vi "ActionVIOnCompile.vi"(8 "error in (no error)":errorcluster, 11 "Device Item Ref in":T1 format="%.0x") -> (0 "error out":errorcluster)   [LabVIEW 2023, in "Embedded TDMS Logger System Explorer.lvlib"]
uses:
  Embedded TDMS Logger System Explorer.lvlib
  <vilib>/NI VeriStand/Custom Device API/Custom Device Item Ref.ctl
  Shared/Compiled.Settings.ctl
  Shared/FileData.ctl
  Shared/GroupData.ctl
  Shared/Meta Data Item.ctl
  Shared/ChannelData.ctl
  <vilib>/NI VeriStand/Custom Device API/Data Reference.ctl
  Shared/SegmentOptions.ctl
  <vilib>/NI VeriStand/Custom Device API/Custom Device Channel Type.ctl
  <vilib>/NI VeriStand/Custom Device API/Get Item Property (U16).vi
  <vilib>/NI VeriStand/Custom Device API/Get Item Property (Variant).vi
  <vilib>/NI VeriStand/Custom Device API/Get Item Property (Dependent Node Pointer).vi
  <vilib>/NI VeriStand/Custom Device API/Get Item Property (Boolean).vi
  <vilib>/NI VeriStand/Custom Device API/Get Item Property (String).vi
  <vilib>/NI VeriStand/Custom Device API/Get Item Property (Double).vi
  <vilib>/NI VeriStand/Custom Device API/Set Item Property (Variant).vi
  <vilib>/NI VeriStand/Custom Device API/Custom Device API.lvlib
  <vilib>/NI/NIVS Inline Async API/_Data Access System Explorer/Data Access System Explorer.lvlib
  Shared/Embedded TDMS Logger Shared.lvlib
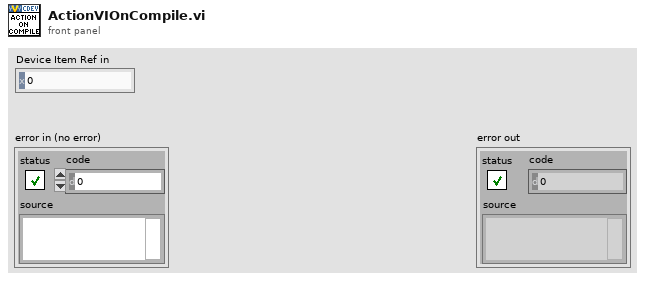
[diagram p1: front panel]
types:
  T1 = typedef "Custom Device API.lvlib/Custom Device Item Ref.ctl" = u64
  T2 = cluster{"Name":string, "Type":enum16{"Output/Write", "Input/Read", "Input/ReadWrite"}, "VS Refs":T1[]}
  T3 = enum16{"Output/Write", "Input/Read", "Input/ReadWrite"}
  T4 = typedef "Custom Device API.lvlib/Custom Device Channel Type.ctl" = enum16{"Input", "Output"}
  T5 = typedef "Embedded TDMS Logger Shared.lvlib/FileData.ctl" = cluster{"Date Captured":string, "Directory":string, "Name":string, "Groups":T6[], "Meta Data":T7[]}
  T6 = typedef "Embedded TDMS Logger Shared.lvlib/GroupData.ctl" = cluster{"Data Rate":string, "Meta Data":T7[], "Channels":T8[], "Name":string}
  T7 = typedef "Embedded TDMS Logger Shared.lvlib/Meta Data Item.ctl" = cluster{"Key":string, "Value":string}
  T8 = typedef "Embedded TDMS Logger Shared.lvlib/ChannelData.ctl" = cluster{"Name":string, "Meta Data":T7[], "Data Reference":T9, "Wfm?":bool, "Increment":dbl}
  T9 = typedef "Custom Device API.lvlib/Data Reference.ctl" = i32
  T10 = typedef "Embedded TDMS Logger Shared.lvlib/Compiled.Settings.ctl" = cluster{"Name":string, "Async Init Timeout":u16, "File Data":T5, "Segment Files":bool, "Segment Every":dbl, "Trigger?":bool, "Segment by":T11, "Trigger Ref":T9}
  T11 = typedef "SegmentOptions.ctl" = enum16{"Time (s)", "Size (MB)"}
  T12 = typedef "Custom Device API.lvlib/Custom Device Item Info.ctl" = cluster{"Name":string, "Is Channel":bool, "GUID":string, "Is Waveform":bool}
  T13 = typedef "Custom Device API.lvlib/Waveform Data Reference.ctl" = i32
  T14 = cluster{"Name":string, "Type":enum16{"Output/Write", "Input/Read", "Input/ReadWrite"}, "VS Refs":T1[]}[]
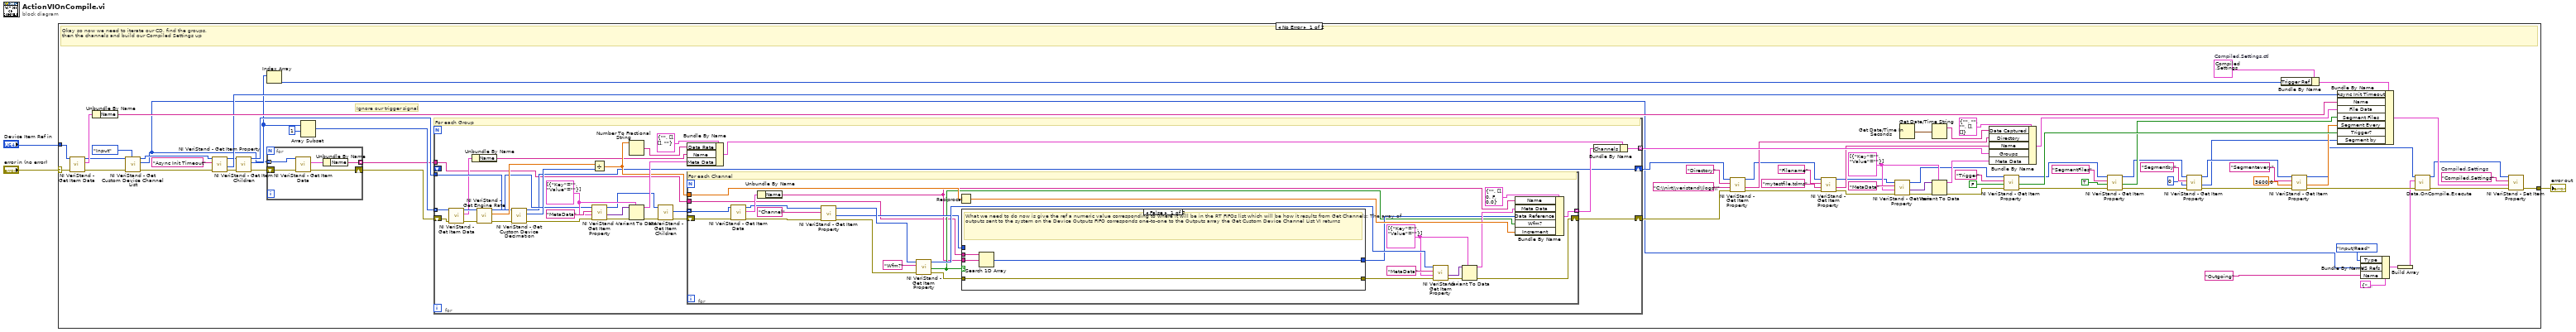
[diagram p0: block diagram]
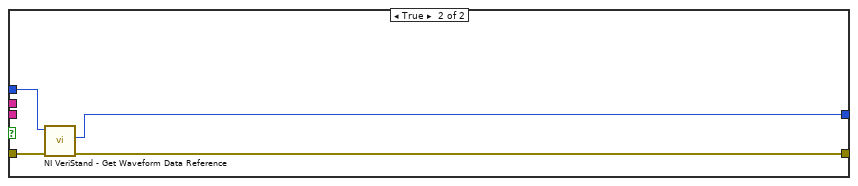
[diagram p2: hidden frame]
diagram:
  n1 = case shown="No Error" "error in (no error)" {
    selector: "error in (no error)" -> [w78 w152]
    tunnel: [w79 w152] -> w2
    tunnel: "Device Item Ref in" -> [w65 _]
    frame No Error {
      w42 = T7[] [{"Key"="", "Value"=""}]
      w50 = T10 {"Name"="", "Async Init Timeout"=0, "File Data"={"Date Captured"="", "Directory"="", "Name"="", "Groups"=[], "Meta Data"=[]}, "Segment Files"=FALSE, "Segment Every"=0.0, "Trigger?"=FALSE, "Segment by"=enum."Size (MB)", "Trigger Ref"=0}  # Compiled.Settings.ctl
      w81 = "Compiled.Settings"  # Compiled.Settings
      # "Ignore our trigger signal"
      # "Okay so now we need to iterate our CD, find the groups,\nthen the channels and build our Compiled Settings up"
      n2 = call <vilib>:"NI VeriStand - Get Item Data.vi"("error in (no error)"=w78, "Item Ref in"=w65) -> ("error out"=w17:errorcluster, "Item Info"=w77:T12, "Item Ref out"=w18:T1)  [unwired: 6 in, 1 out]
      n3 = Unbundle By Name(w77) -> ("Name"=w76:string)
      n4 = call <vilib>:"NI VeriStand - Get Custom Device Channel List.vi"("Channel Type"=Custom_Device_Channel_Type."Input", "error in (no error)"=w17, "Device Ref in"=w18) -> ("error out"=w16:errorcluster, "Specified Channel Ref List"=w7:T1[], "Device Ref out"=w15:T1)  [unwired: 6 in]
      n5 = call-poly <vilib>:"NI VeriStand - Get Item Property.vi"("error in (no error)"=w16, "Property Name"="Async Init Timeout", "Item Ref in"=w15) -> ("error out"=w71:errorcluster, "Value"=w72:u16, "Item Ref out"=w58:T1)  [unwired: 5 in, 1 out]
      n6 = call <vilib>:"NI VeriStand - Get Item Children.vi"("error in (no error)"=w71, "Item Ref in"=w58) -> ("error out"=w13:errorcluster, "Child Refs"=w51:T1[], "Item Ref out"=w56:T1)  [unwired: 6 in, 1 out]
      n7 = Index Array(array=w51) -> (element=w49:T1)  [unwired: 1 in]
      n8 = for {
        tunnel: w7 -> [w86] mode=indexing
        tunnel: [w84] -> w14 mode=indexing
        shift-right: [w83] -> w12
        shift-left: w13 -> [w82]
        n9 = call <vilib>:"NI VeriStand - Get Item Data.vi"("error in (no error)"=w82, "Item Ref in"=w86) -> ("error out"=w83:errorcluster, "Item Info"=w85:T12)  [unwired: 8 out]
        n10 = Unbundle By Name(w85) -> ("Name"=w84:string)
      }
      n11 = Array Subset(array=w51, index=1 ("length")) -> (w55:T1[])  [unwired: 1 in]
      n12 = for {
        tunnel: w55 -> [w94] mode=indexing
        shift-right: [w97] -> w60
        shift-left: w12 -> [w93]
        tunnel: [w115] -> w69 mode=indexing
        tunnel: w56 -> [w107]
        shift-right: [w88] -> w59
        shift-left: _ -> [_]
        tunnel: w14 -> [w87]
        w104 = T7[] [{"Key"="", "Value"=""}]
        # "For each Group"
        n13 = call <vilib>:"NI VeriStand - Get Item Data.vi"("error in (no error)"=w93, "Item Ref in"=w94) -> ("error out"=w92:errorcluster, "Item Info"=w90:T12, "Item Ref out"=w91:T1)  [unwired: 7 out]
        n14 = Unbundle By Name(w90) -> ("Name"=w89:string)
        n15 = call <vilib>:"NI VeriStand - Get Engine Rate.vi"("error in (no error)"=w92, "Item Ref in"=w91) -> ("error out"=w108:errorcluster, "Rate (Hz)"=w111:dbl, "Item Ref out"=w96:T1)  [unwired: 7 in]
        n16 = call <vilib>:"NI VeriStand - Get Custom Device Decimation.vi"("error in (no error)"=w108, "Device Ref in"=w107) -> ("error out"=w102:errorcluster, "Decimation"=w110:i32, "Device Ref out"=w88:T1)  [unwired: 7 in]
        n17 = Divide(x=w111, y=w110) -> (x/y=w99:dbl)
        n18 = call-poly <vilib>:"NI VeriStand - Get Item Property.vi"("error in (no error)"=w102, "Default Value"=w104, "Property Name"="MetaData", "Item Ref in"=w96) -> ("error out"=w101:errorcluster, "Value"=w105:variant, "Item Ref out"=w95:T1)  [unwired: 4 in, 1 out]
        n19 = Number To Fractional String(number=w99) -> (F-format string=w109:string)  [unwired: 3 in]
        n20 = Variant To Data(error in=w101, type=w104, Variant=w105) -> (data=w103:T7[], error out=w100:errorcluster)
        n21 = call <vilib>:"NI VeriStand - Get Item Children.vi"("error in (no error)"=w100, "Item Ref in"=w95) -> ("error out"=w98:errorcluster, "Child Refs"=w112:T1[])  [unwired: 6 in, 2 out]
        n22 = Bundle By Name(cluster=T6 {"Data Rate"="", "Meta Data"=[], "Channels"=[], "Name"=""} ("Group Data"), "Data Rate"=w109, "Name"=w89, "Meta Data"=w103) -> (w113:T6)
        n23 = for {
          tunnel: [w142] -> w116 mode=indexing
          tunnel: w112 -> [w125] mode=indexing
          tunnel: w99 -> [w140]
          shift-right: [w129] -> w97
          shift-left: w98 -> [w124]
          tunnel: w87 -> [w117]
          w131 = T7[] [{"Key"="", "Value"=""}]
          # "For each Channel"
          n24 = call <vilib>:"NI VeriStand - Get Item Data.vi"("error in (no error)"=w124, "Item Ref in"=w125) -> ("error out"=w128:errorcluster, "Item Info"=w127:T12, "Item Ref out"=w126:T1)  [unwired: 7 out]
          n25 = Unbundle By Name(w127) -> ("Name"=w118:string)
          n26 = call-poly <vilib>:"NI VeriStand - Get Item Property.vi"("error in (no error)"=w128, "Property Name"="Channel", "Item Ref in"=w126) -> ("error out"=w136:errorcluster, "Dependent Node Ref"=w123:T1, "Item Ref out"=w137:T1)  [unwired: 5 in, 1 out]
          n27 = call-poly <vilib>:"NI VeriStand - Get Item Property.vi"("error in (no error)"=w136, "Property Name"="Wfm?", "Item Ref in"=w137) -> ("error out"=w122:errorcluster, "Value"=w119:bool, "Item Ref out"=w134:T1)  [unwired: 5 in, 1 out]
          n28 = Reciprocal(x=w140) -> (1/x=w141:dbl)
          n29 = case shown="False" w119 {
            tunnel: w123 -> [_ w151]
            tunnel: w122 -> [w147 w150]
            tunnel: [w147 w149] -> w121
            tunnel: [w144 w148] -> w120
            tunnel: w118 -> [w146 _]
            tunnel: w117 -> [w145 _]
            frame False {
              # "What we need to do now is give the ref a numeric value corresponding to where it will be in the RT FIFOs list which will be how it results from Get Channels: The array of outputs sent to the system on the Device Outputs FIFO corresponds one-to-one to the Outputs array the Get Custom Device Channel List VI returns"
              n30 = Search 1D Array(1D array=w145, element=w146) -> (index of element=w144:i32)  [unwired: 1 in]
            }
            frame True {
              n31 = call <vilib>:"NI VeriStand - Get Waveform Data Reference.vi"("error in (no error)"=w150, "Waveform Ref in"=w151) -> ("error out"=w149:errorcluster, "Waveform Data Reference"=w148:T13)  [unwired: 7 in, 1 out]
            }
          }
          n32 = call-poly <vilib>:"NI VeriStand - Get Item Property.vi"("error in (no error)"=w121, "Default Value"=w131, "Property Name"="MetaData", "Item Ref in"=w134) -> ("error out"=w133:errorcluster, "Value"=w132:variant)  [unwired: 4 in, 2 out]
          n33 = Variant To Data(error in=w133, type=w131, Variant=w132) -> (data=w130:T7[], error out=w129:errorcluster)
          n34 = Bundle By Name(cluster=T8 {"Name"="", "Meta Data"=[], "Data Reference"=0, "Wfm?"=FALSE, "Increment"=0.0} ("Channel Data"), "Name"=w118, "Meta Data"=w130, "Data Reference"=w120, "Wfm?"=w119, "Increment"=w141) -> (w142:T8)
        }
        n35 = Bundle By Name(cluster=w113, "Channels"=w116) -> (w115:T6)
      }
      n36 = call-poly <vilib>:"NI VeriStand - Get Item Property.vi"("error in (no error)"=w60, "Default Value"="C:\\nirt\\veristand\\logs\\", "Property Name"="Directory", "Item Ref in"=w59) -> ("error out"=w46:errorcluster, "Value"=w64:string, "Item Ref out"=w61:T1)  [unwired: 4 in, 1 out]
      n37 = call-poly <vilib>:"NI VeriStand - Get Item Property.vi"("error in (no error)"=w46, "Default Value"="mytestfile.tdms", "Property Name"="Filename", "Item Ref in"=w61) -> ("error out"=w44:errorcluster, "Value"=w57:string, "Item Ref out"=w41:T1)  [unwired: 4 in, 1 out]
      n38 = call-poly <vilib>:"NI VeriStand - Get Item Property.vi"("error in (no error)"=w44, "Default Value"=w42, "Property Name"="MetaData", "Item Ref in"=w41) -> ("error out"=w43:errorcluster, "Value"=w45:variant, "Item Ref out"=w37:T1)  [unwired: 4 in, 1 out]
      n39 = Get Date/Time In Seconds() -> (seconds since 1Jan1904=w53:timestamp)
      n40 = Get Date/Time String(seconds (now)=w53) -> (date string=w52:string)  [unwired: 2 in, 1 out]
      n41 = Variant To Data(error in=w43, type=w42, Variant=w45) -> (data=w40:T7[], error out=w36:errorcluster)
      n42 = Bundle By Name(cluster=T5 {"Date Captured"="", "Directory"="", "Name"="", "Groups"=[], "Meta Data"=[]} ("File Data"), "Date Captured"=w52, "Directory"=w64, "Name"=w57, "Groups"=w69, "Meta Data"=w40) -> (w68:T5)
      n43 = call-poly <vilib>:"NI VeriStand - Get Item Property.vi"("error in (no error)"=w36, "Default Value"=FALSE, "Property Name"="Trigger", "Item Ref in"=w37) -> ("error out"=w33:errorcluster, "Value"=w35:bool, "Item Ref out"=w34:T1)  [unwired: 4 in, 1 out]
      n44 = call-poly <vilib>:"NI VeriStand - Get Item Property.vi"("error in (no error)"=w33, "Default Value"=TRUE, "Property Name"="SegmentFiles", "Item Ref in"=w34) -> ("error out"=w29:errorcluster, "Value"=w30:bool, "Item Ref out"=w28:T1)  [unwired: 4 in, 1 out]
      n45 = call-poly <vilib>:"NI VeriStand - Get Item Property.vi"("error in (no error)"=w29, "Default Value"=u16 0, "Property Name"="Segmentby", "Item Ref in"=w28) -> ("error out"=w23:errorcluster, "Value"=w19:u16, "Item Ref out"=w22:T1)  [unwired: 4 in, 1 out]
      n46 = Bundle By Name(cluster=w50, "Trigger Ref"=w49) -> (w48:T10)
      n47 = call-poly <vilib>:"NI VeriStand - Get Item Property.vi"("error in (no error)"=w23, "Default Value"=3600.0, "Property Name"="Segmentevery", "Item Ref in"=w22) -> ("error out"=w21:errorcluster, "Value"=w20:dbl, "Item Ref out"=w6:T1)  [unwired: 4 in, 1 out]
      n48 = Bundle By Name(cluster=w48, "Async Init Timeout"=w72, "Name"=w76, "File Data"=w68, "Segment Files"=w30, "Segment Every"=w20, "Trigger?"=w35, "Segment by"=w19) -> (w80:T10)
      n49 = Bundle By Name(cluster=T2 {"Name"="", "Type"=enum."Output/Write", "VS Refs"=[]} ("Group"), "Type"=T3."Input/Read", "VS Refs"=w7, "Name"="Outgoing" ("Item Name")) -> (w5:T2)
      n50 = Build Array(w5) -> (w4:T14)
      n51 = call <vilib>:"Data.OnCompile.Execute.vi"("error in"=w21, "VS Ref Groups"=w4, "Custom Device Ref"=w6) -> ("error out"=w75:errorcluster, "Custom Device Ref"=w74:T1)  [unwired: 7 in]
      n52 = call-poly <vilib>:"NI VeriStand - Set Item Property.vi"("error in (no error)"=w75, "Value"=w80, "Property Name"=w81, "Item Ref in"=w74) -> ("error out"=w79:errorcluster)  [unwired: 5 in, 2 out]
    }
    frame Error {
    }
  }
  "error out" <- w2
